vi "NT Read Numeric Array.vi"(4 "options":T1={"Send All"=FALSE, "Keep Duplicates"=FALSE, "rate (hz)"=10}, 8 "error in":errorcluster, 9 "default value":dbl[](array[numeric]), 11 "name":string="Number Array") -> (0 "error out":errorcluster, 1 "timestamp":u64, 3 "value":dbl[](array[numeric]))   [LabVIEW 2025]
doc: "Return the double precision numeric array data stored in the named topic. Returns an error and the default value if topic not present."
uses:
  <vilib>/Rock Robotics/Network Tables/NT SubscribeOptions.ctl
  <vilib>/Rock Robotics/Network Tables/NT Datatype.ctl
panel:
  in  "description":string="double[]"
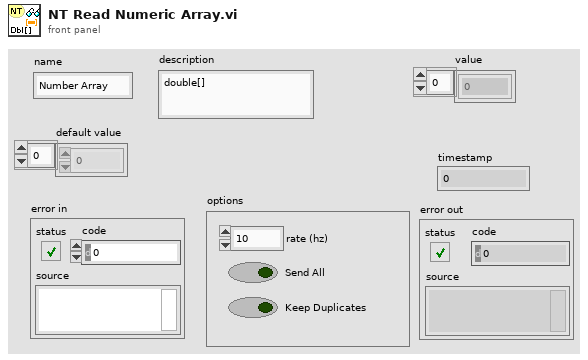
[diagram p1: front panel]
types:
  T1 = typedef "NT SubscribeOptions.ctl" = cluster{"Send All":bool, "Keep Duplicates":bool, "rate (hz)":u64}
  T2 = typedef "NT Datatype.ctl" = u32
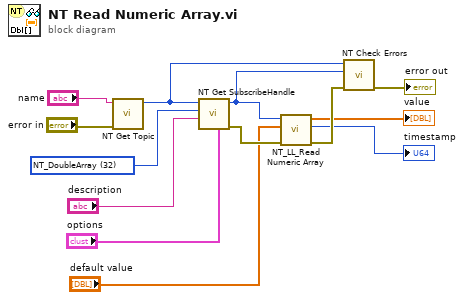
[diagram p0: block diagram]
diagram:
  w6 = T2 32 items=["NT_Unassigned"=0, "NT_Boolean"=1, "NT_Double"=2, "NT_String"=4, "NT_Raw"=8, "NT_BooleanArray"=16, "NT_DoubleArray"=32, "NT_StringArray"=64, "NT_RPC"=128, "NT_Integer"=256, "NT_Float"=512, "NT_IntegerArray"=1024, "NT_FloatArray"=2048] ("NT_Type")
  n1 = call <vilib>:"NT Get Topic.vi"("error in (no error)"="error in", "name"="name") -> ("topicHandle"=w10:u32)  [unwired: 8 in, 1 out]
  n2 = call <vilib>:"NT Get SubscribeHandle.vi"("options"="options", "description"="description", "NT_Type"=w6, "topicHandle"=w10) -> ("error out"=w8:errorcluster, "subscribeHandle"=w7:u32)  [unwired: 6 in]
  n3 = call <vilib>:"NT_LL_Read Numeric Array.vi"("error in (no error)"=w8, "default value"="default value", "subscribeHandle"=w7) -> ("error out"=w9:errorcluster, "time"=→"timestamp":i64, "value"=→"value":dbl[])  [unwired: 6 in]
  n4 = call <vilib>:"NT Check Errors.vi"("error in (no error)"=w9, "pubSubHandle"=w7, "topicHandle"=w10) -> ("error out"=→"error out":errorcluster)  [unwired: 8 in]
